vi "Serial_Logging_Global.vi"() -> ()   [LabVIEW 2010]
panel:
  in  "Commands to log (Default All)":string[](array[string])
  in  "Log Array3":string[](array[string])
  in  "Log Array2":string[](array[string])
  in  "Log Array1":string[](array[string])
  in  "Channels to Log":string[](array[string])
  in  "Serial Logging":bool
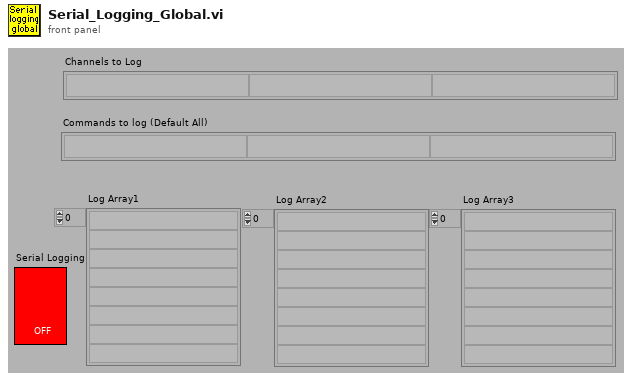
[diagram p1: front panel]
diagram:
